vi "reconnect to error stream delayed message.vi"(8 "error in (no error)":errorcluster, 11 "RT Queues":T1) -> ()   [LabVIEW 2018]
uses:
  Type Defs/Queues cluster.ctl
  ICL-LabVIEW_General/Message Scheduler/message scheduler.lvclass
  Queue VIs/En-queue RT comms element.vi
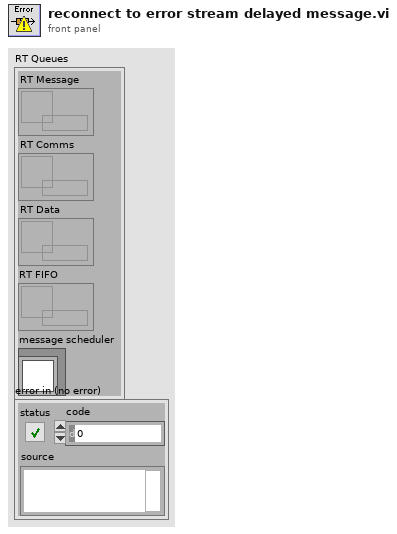
[diagram p1: front panel]
types:
  T1 = typedef "Queues cluster.ctl" = cluster{"RT Message":refnum<queue>, "RT Comms":refnum<queue>, "RT Data":refnum<queue>, "RT FIFO":refnum<queue>, "message scheduler":refnum<class "message scheduler.lvclass">}
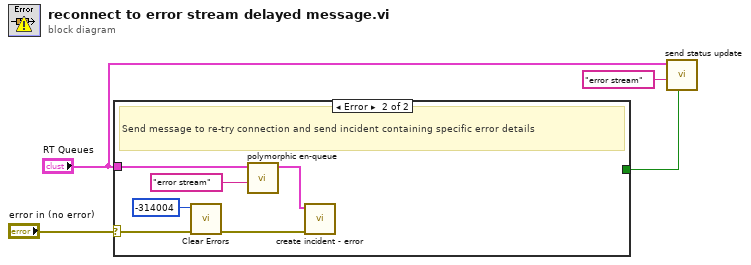
[diagram p0: block diagram]
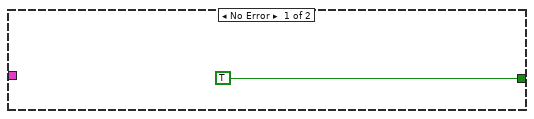
[diagram p2: hidden frame]
diagram:
  n1 = case shown="Error" "error in (no error)" {
    selector: "error in (no error)" -> [_ w8]
    tunnel: "RT Queues" -> [_ w10]
    tunnel: [TRUE _] -> w1
    frame No Error {
    }
    frame Error {
      # "Send message to re-try connection and send incident containing specific error details"
      n2 = call <vilib>:"Clear Errors.vi"("error in (no error)"=w8, "specific error code to clear (0: all)"=-314004) -> ("error out"=w7:errorcluster)  [unwired: 4 in, 1 out]
      n3 = call-poly "polymorphic en-queue.vi"("Message"="error stream" ("message"), "RT Queues"=w10) -> ("RT Queues out"=w6:T1)  [unwired: 9 in]
      n4 = call "create incident - error.vi"("error"=w7, "RT Queues"=w6) -> ()  [unwired: 9 in, 1 out]
    }
  }
  n5 = call "send status update.vi"("status (F)"=w1, "subject"="error stream" ("Message"), "RT Queues"="RT Queues") -> ()  [unwired: 8 in, 1 out]
